vi "Write SAP Wav.vi"(8 "error in (no error)":errorcluster, 9 "Audio Size ( bytes)":i32, 10 "input cluster":T1={"sound quality"=enum."mono", "bits per sample"=enum."16 bit", "rate"=8000} {"rate" min=4000 step=1000}, 11 "wave file path":path) -> (0 "error out":errorcluster, 3 "wave file path out":path)   [LabVIEW 2016]
doc: "Stores waveform data and its sound format information into a file."
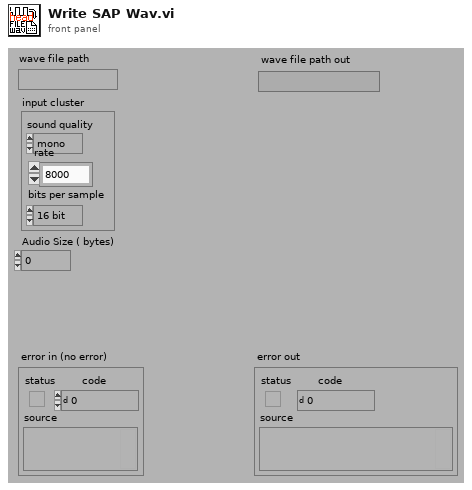
[diagram p1: front panel]
types:
  T1 = cluster{"sound quality":enum16{"mono", "stereo"}, "bits per sample":enum16{"8 bit", "16 bit"}, "rate":u32}
  T2 = enum16{"read/write", "read-only", "write-only", "write-only (truncate)"}
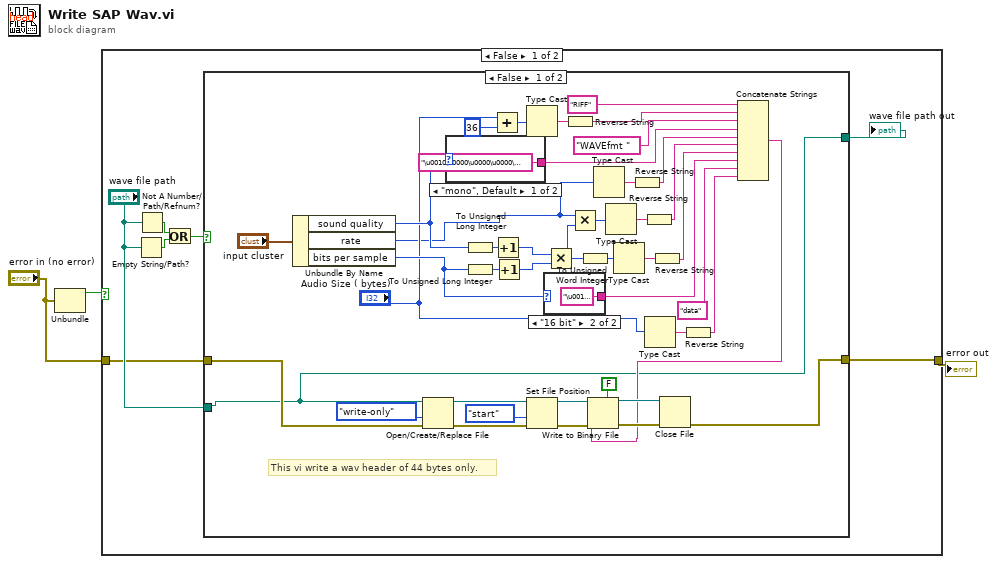
[diagram p0: block diagram]
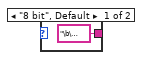
[diagram p2: hidden frame]
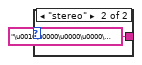
[diagram p3: hidden frame]
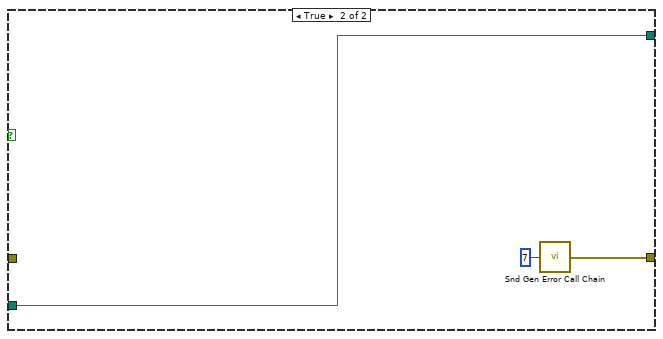
[diagram p4: hidden frame]
diagram:
  n1 = Unbundle("error in (no error)") -> ("status"=w1:bool)  [unwired: 2 out]
  n2 = case shown="False" w1 {
    tunnel: [w4 w60] -> w3
    tunnel: "error in (no error)" -> [w5 w60]
    frame False {
      n3 = Empty String/Path?(string/path="wave file path") -> (empty?=w9:bool)
      n4 = Not A Number/Path/Refnum?(number/path/refnum="wave file path") -> (NaN/Path/Refnum?=w10:bool)
      n5 = Or(x=w10, y=w9) -> (x .or. y?=w8:bool)
      n6 = case shown="False" w8 {
        tunnel: "wave file path" -> [w15 w59]
        tunnel: [w15 w59] -> w6
        tunnel: [w18 w57] -> w4
        tunnel: w5 -> [w21 _]
        frame False {
          # "This vi write a wav header of 44 bytes only."
          n7 = Unbundle By Name("input cluster") -> ("sound quality"=w28:enum16{"mono", "stereo"}, "rate"=w14:u32, "bits per sample"=w27:enum16{"8 bit", "16 bit"})
          n8 = Open/Create/Replace File(file path (use dialog)=w15, error in=w21, access (0:read/write)=T2."write-only" ("open mode (0)")) -> (refnum out=w23:refnum<file>, error out=w20:errorcluster)  [unwired: 4 out]
          n9 = case shown="\"mono\", Default" w28 {
            tunnel: ["\u0010\u0000\u0000\u0000\u0001\u0000\u0001\u0000" "\u0010\u0000\u0000\u0000\u0001\u0000\u0002\u0000"] -> w29
            frame "mono", Default {
            }
            frame "stereo" {
            }
          }
          n10 = To Unsigned Long Integer(number=w28) -> (unsigned 32bit integer=w40:u32)
          n11 = To Unsigned Long Integer(number=w27) -> (unsigned 32bit integer=w39:u32)
          n12 = Add(x="Audio Size ( bytes)", y=36) -> (x+y=w47:i32)
          n13 = Increment(x=w40) -> (x+1=w38:u32)
          n14 = Increment(x=w39) -> (x+1=w37:u32)
          n15 = Type Cast(x=w47) -> (*(type *) &x=w49:string)  [unwired: 1 out]
          n16 = Set File Position(refnum=w23, from (0:start)=enum16{"start", "end", "current"}."start" ("pos mode (0:2)"), error in=w20) -> (refnum out=w13:refnum<file>, error out=w12:errorcluster)  [unwired: 1 out]
          n17 = case shown="\"16 bit\"" w27 {
            tunnel: ["\b\u0000" "\u0010\u0000"] -> w26
            frame "8 bit", Default {
            }
            frame "16 bit" {
            }
          }
          n18 = Multiply(x=w38, y=w37) -> (x*y=w35:u32)
          n19 = Reverse String(1:w49) -> (0:w46:string)
          n20 = Multiply(x=w14, y=w35) -> (x*y=w41:u32)
          n21 = To Unsigned Word Integer(number=w35) -> (unsigned 16bit integer=w34:u16)
          n22 = Type Cast(x=w14) -> (*(type *) &x=w45:string)  [unwired: 1 out]
          n23 = Type Cast(x=w41) -> (*(type *) &x=w43:string)  [unwired: 1 out]
          n24 = Type Cast(x=w34) -> (*(type *) &x=w36:string)  [unwired: 1 out]
          n25 = Reverse String(1:w45) -> (0:w44:string)
          n26 = Reverse String(1:w43) -> (0:w42:string)
          n27 = Type Cast(x="Audio Size ( bytes)") -> (*(type *) &x=w50:string)  [unwired: 1 out]
          n28 = Reverse String(1:w36) -> (0:w33:string)
          n29 = Reverse String(1:w50) -> (0:w31:string)
          n30 = Concatenate Strings("RIFF", w46, "WAVEfmt ", w29, w44, w42, w33, w26, "data", w31) -> (w17:string)
          n31 = Write to Binary File(file (use dialog)=w13, data=w17, error in=w12, 5:FALSE ("prepend array or string size? (T)")) -> (refnum out=w22:refnum<file>, error out=w19:errorcluster)  [unwired: 3 out]
          n32 = Close File(refnum=w22, error in=w19) -> (error out=w18:errorcluster)  [unwired: 1 out]
        }
        frame True {
          n33 = call <vilib>:"Snd Gen Error Call Chain.vi"("error code"=7) -> ("error out"=w57:errorcluster)
        }
      }
      "wave file path out" <- w6
    }
    frame True {
    }
  }
  "error out" <- w3
